vi "Test Sec-WebSocket-Key.vi"() -> ()   [LabVIEW 2020]
uses:
  Crypto/SHA-1/SHA-1.lvclass
  lv-base64/Base64.lvlib
panel:
  out "Sec-WebSocket-Accept":string
  in  "Sec-WebSocket-Key":string="dGhlIHNhbXBsZSBub25jZQ=="
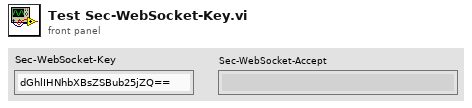
[diagram p1: front panel]
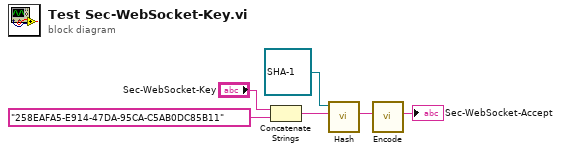
[diagram p0: block diagram]
diagram:
  n1 = Concatenate Strings("Sec-WebSocket-Key", "258EAFA5-E914-47DA-95CA-C5AB0DC85B11" ("string")) -> (w4:string)
  n2 = call-dynamic "Hash.vi"("Message"=w4, "SHA-1 in"=refnum<class "SHA-1.lvclass"> refnum) -> ("Hash"=w2:string)  [unwired: 7 in, 2 out]
  n3 = call "Encode.vi"("string in (not encoded)"=w2) -> ("string out (base64-encoded)"=→"Sec-WebSocket-Accept":string)  [unwired: 9 in, 1 out]
